vi "DF PROFINET IO GettingStarted Controller.vi"() -> ()   [LabVIEW 2019]
doc: "This VI shows how configured PROFINET devices can be accessed with a KUNBUS DF PROFINET IO interface card as Controller."
uses:
  <vilib>/KUNBUS GmbH/DF PROFINET IO/CS_PN_Profinet_StartStopMode.ctl
  <vilib>/KUNBUS GmbH/DF PROFINET IO/CS_PN_Controller_StartStopMode.ctl
  <vilib>/KUNBUS GmbH/DF PROFINET IO/CS_PN_Controller_WriteRecordReq.ctl
  <vilib>/KUNBUS GmbH/DF PROFINET IO/CS_PN_Controller_ReadRecordReq.ctl
  <vilib>/KUNBUS GmbH/DF PROFINET IO/CS_PN_Controller_AlarmClass.ctl
  <vilib>/Utility/error.llb/DialogType.ctl
panel:
  in  "Update time":u32=1 caption="(ms)"
  in  "Tab Control":enum32{"Process Data", "Read/Write Record Data"}(tab)
  out "Output data:":string
  out "Input data:":string
  in  "Modify output data:":string
  in  "Device List":i32(listbox)
  in  "Set output data":bool
  out "Description:":string
  in  "Get diagnostic data":bool
  in  "Get process data":bool
  in  "APDU status:":bool
  in  "Device status:":bool
  in  "Get modulediffblock":bool
  out "APDU status":u8 format="0x%02x"
  out "APDU status:":bool
  out "Device status":bool=TRUE
  out "Device status:":u8 format="0x%02x"
  in  "Output status 2":bool=TRUE caption="Status"
  out "Input status 2":u8 format="0x%02x"
  out "Input status":bool
  out "Output status 3":u8 format="0x%02x"
  out "Output status":bool
  out "Read record data:":string
  in  "Write record data:":string
  in  "Write Record":bool
  in  "Read Record":bool
  out "R/W Record Result":string
  out "Error out":errorcluster
  in  "Device":u16
  in  "Slot":u16
  in  "SubSlot":u16
  in  "Timeout":u32
  in  "Read data length":u32
  in  "Index":u16 format="%.0x"
  in  "Stop":bool
  in  "PROFINET Controller":refnum<visa-resource-name>
  # "Instructions:\n1. Read the Getting Started manual: Help >> KUNBUS GmbH >> DF PROFINET IO\n2. The PROFINET configuration needs to be downloaded to the DF PROFINET IO interface card using the configuration tool Configurator III\n3. Choose the DF PROFINET IO interface card from the VISA control \"PROFINET Controller\" and then start the VI"
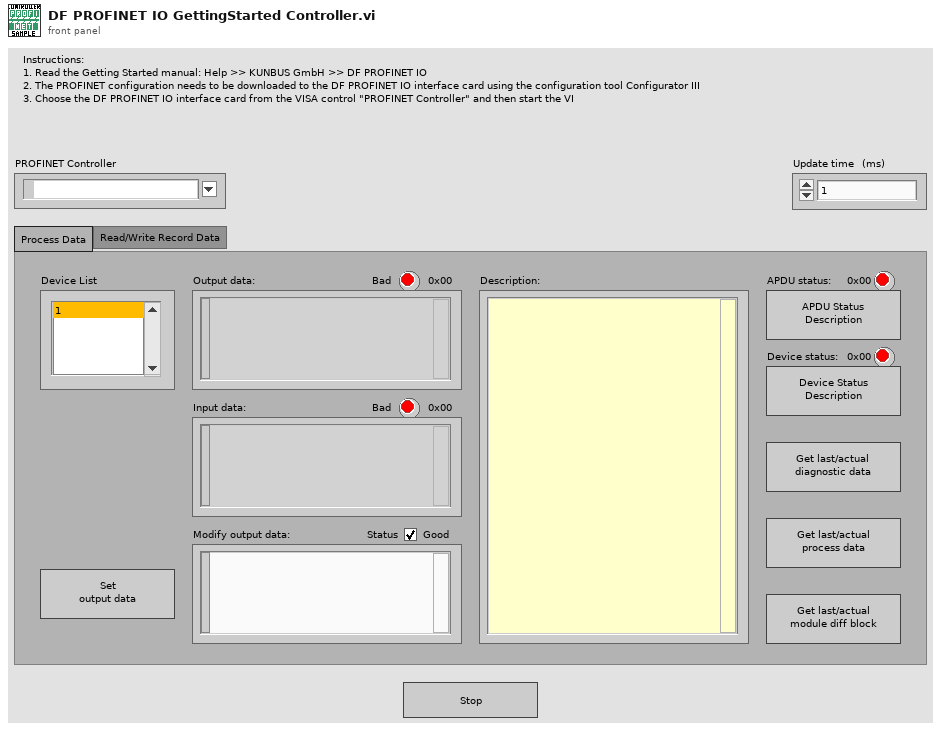
[diagram p1: front panel]
types:
  T1 = typedef "CS_PN_Controller_StartStopMode.ctl" = enum32{"Start Controller", "Stop Controller"}
  T2 = typedef "CS_PN_Profinet_StartStopMode.ctl" = enum32{"Start Controller", "Stop Controller", "Start Device", "Stop Device"}
  T3 = enum16{"APDU status", "Device status", "Diagnostic alarm data", "Process alarm data", "Module diff block"}
  T4 = typedef "CS_PN_Controller_AlarmClass.ctl" = u32
  T5 = typedef "CS_PN_Controller_AlarmData.ctl" = cluster{"Block type:":u16, "Block version:":u16, "Block length:":u16, "Alarm type:":T6, "API:":u32, "Slot number:":u16, "Subslot number:":u16, "Module ident number:":u32, "Submodule ident number:":u32, "Alarm specifier:":u16, "Alarm item:":u8[]}
  T6 = typedef "CS_PN_Controller_AlarmType.ctl" = u16
  T7 = typedef "CS_PN_Controller_ModDiffBlock.ctl" = cluster{"ARID:":u32, "Station name:":string, "Number of modules:":u32, "List of modules":T8[]}
  T8 = typedef "CS_PN_Controller_ModuleDiffBlockSlot.ctl" = cluster{"Slot number:":u32, "Module ident number:":u32, "Module state:":u32, "Number of submodules:":u32, "List of submodules":T9[]}
  T9 = typedef "CS_PN_Controller_ModuleDiffBlockSubslot.ctl" = cluster{"Subslot number:":u32, "Submodule ident number:":u32, "Submodule state:":u32}
  T10 = cluster{"Numeric":i32, "Output status":u8, "unsigned byte array":u8[]}
  T11 = cluster{"Numeric":i32, "Output status":u8, "unsigned byte array":u8[]}[]
  T12 = cluster{"APDU status":u8, "Device status":u8, "Input status":u8, "Input data":u8[], "Output status":u8, "Output data":u8[]}[]
  T13 = cluster{"APDU status":u8, "Device status":u8, "Input status":u8, "Input data":u8[], "Output status":u8, "Output data":u8[]}
  T14 = typedef "DialogType.ctl" = u16
  T15 = typedef "CS_PN_Controller_WriteRecordReq.ctl" = cluster{"Timeout:":u32, "Device:":u16, "Slot number:":u16, "Subslot number:":u16, "Index:":u16, "Record data:":u8[]}
  T16 = typedef "CS_PN_Controller_ReadRecordReq.ctl" = cluster{"Timeout:":u32, "Device:":u16, "Slot number:":u16, "Subslot number:":u16, "Index:":u16, "Data length:":u32}
  T17 = typedef "CS_PN_Controller_WriteRecordRes.ctl" = cluster{"Error code:":u8, "Error decode:":u8, "Error code 1:":u8, "Error code 2:":u8, "Add data 1:":u16, "Add data 2:":u16}
  T18 = typedef "CS_PN_Controller_ReadRecordRes.ctl" = cluster{"Error code:":u8, "Error decode:":u8, "Error code 1:":u8, "Error code 2:":u8, "Add data 1:":u16, "Add data 2:":u16, "Record data:":u8[]}
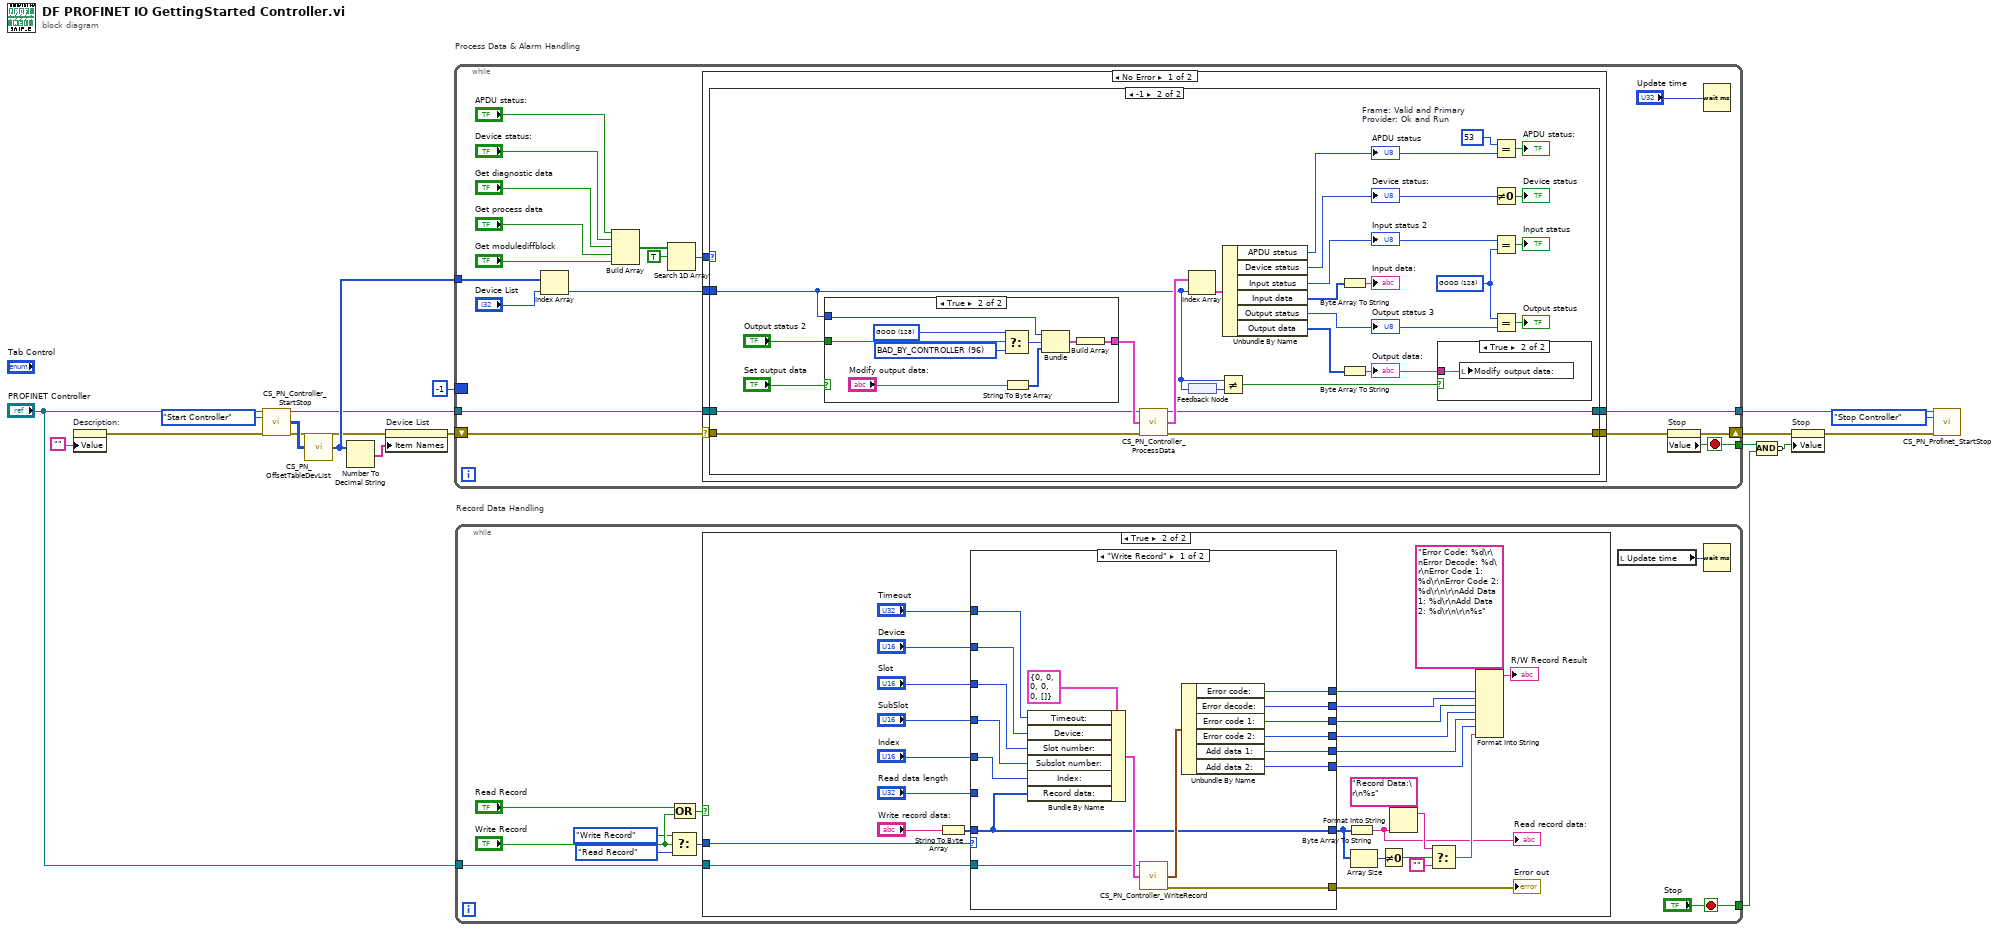
[diagram p0: block diagram]
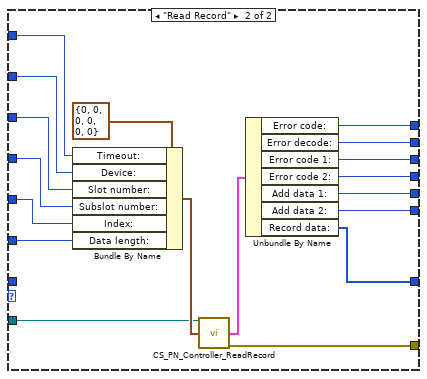
[diagram p3: hidden frame]
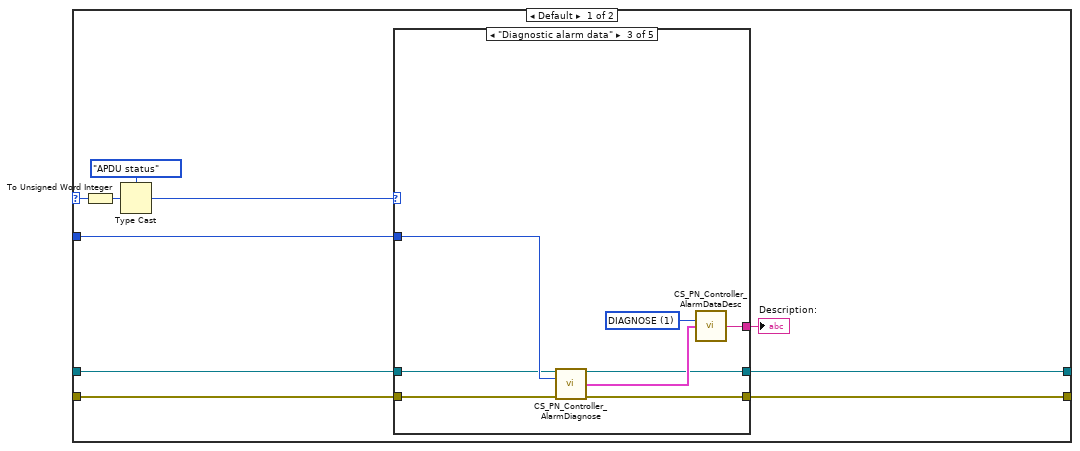
[diagram p4: hidden frame]
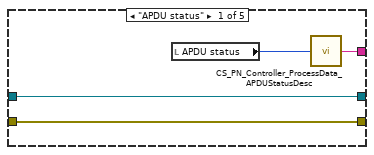
[diagram p5: hidden frame]
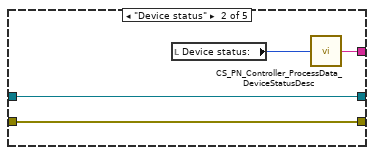
[diagram p6: hidden frame]
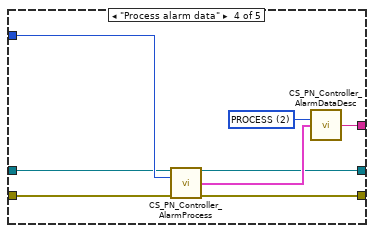
[diagram p7: hidden frame]
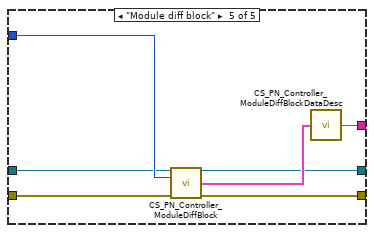
[diagram p8: hidden frame]
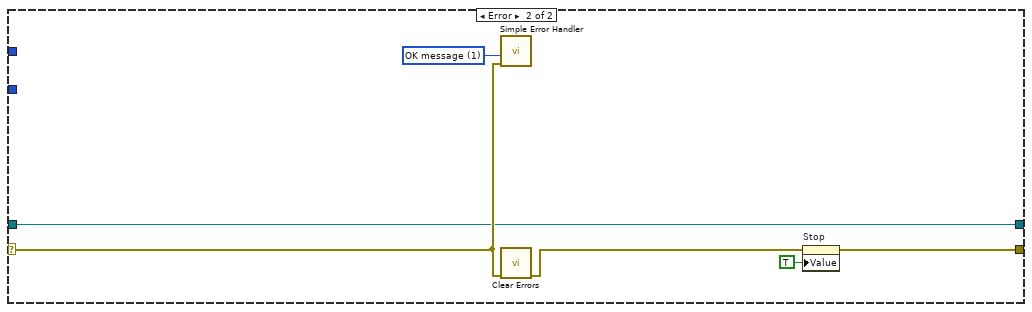
[diagram p11: hidden frame]
diagram:
  n1 = property on="Description:" class="Str"("Value"="") -> (error out=w9:errorcluster)  [unwired: 2 in, 1 out]
  n2 = call <vilib>:"CS_PN_Controller_StartStop.vi"("PN-Controller resource name"="PROFINET Controller", "Mode"=CS_PN_Controller_StartStopMode."Start Controller", "Error In"=w9) -> ("PN-Controller resource name out"=w7:refnum<visa-resource-name>, "Offset table info"=w13:i32[][], "Error Out"=w11:errorcluster)  [unwired: 9 in, 1 out]
  n3 = call <vilib>:"CS_PN_OffsetTableDevList.vi"("Offset table info"=w13) -> ("Device list"=w18:i32[])  [unwired: 14 in]
  n4 = Number To Decimal String(number=w18) -> (decimal integer string=w16:string[])  [unwired: 1 in]
  n5 = property on="Device List" class="LstBox (strict)"(error in=w11, "Item Names"=w16) -> (error out=w10:errorcluster)  [unwired: 1 in, 1 out]
  n6 = while "Process Data & Alarm Handling" {
    tunnel: w7 -> [w25]
    tunnel: [w35] -> w17
    tunnel: w18 -> [w36]
    border: -1 ("InitModifyOutputDataControl") -> [_]
    shift-right: [w20] -> w6
    shift-left: w10 -> [w22]
    tunnel: [w19] -> w3
    stop <- w19 stop-if-true
    n7 = Index Array(array=w36, index="Device List") -> (element=w34:i32)
    n8 = Build Array("APDU status:", "Device status:", "Get diagnostic data", "Get process data", "Get modulediffblock") -> (w30:bool[])
    n9 = Search 1D Array(1D array=w30, element=TRUE) -> (index of element=w24:i32)  [unwired: 1 in]
    n10 = case shown="No Error" w22 {
      selector: w22 -> [w37 w125]
      tunnel: [w42 w124] -> w35
      tunnel: w34 -> [w41 _]
      tunnel: w25 -> [w40 w124]
      tunnel: w24 -> [w39 _]
      tunnel: [w38 w122] -> w21
      frame No Error {
        n11 = case shown="-1" w39 {
          selector: w39 -> [w45 _]
          tunnel: w37 -> [w46 w109]
          tunnel: w40 -> [w47 w86]
          tunnel: [w43 w108] -> w38
          tunnel: [w44 w85] -> w42
          tunnel: w41 -> [w48 w87]
          frame Default {
            n12 = To Unsigned Word Integer(number=w45) -> (unsigned 16bit integer=w50:u16)
            n13 = Type Cast(type=T3."APDU status", x=w50) -> (*(type *) &x=w51:T3)
            n14 = case shown="\"Diagnostic alarm data\"" w51 {
              tunnel: w46 -> [w56 w59 w67 w75 w80]
              tunnel: w47 -> [w55 w60 w61 w74 w81]
              tunnel: [w56 w59 w65 w73 w79] -> w43
              tunnel: w48 -> [_ _ w68 w76 w83]
              tunnel: [w54 w58 w64 w71 w78] -> w52
              tunnel: [w55 w60 w63 w70 w77] -> w44
              frame "APDU status" {
                n15 = local read "APDU status"() -> (w53:u8)
                n16 = call <vilib>:"CS_PN_Controller_ProcessData_APDUStatusDesc.vi"("APDU Status"=w53) -> ("Description:"=w54:string)  [unwired: 14 in]
              }
              frame "Device status" {
                n17 = local read "Device status:"() -> (w57:u8)
                n18 = call <vilib>:"CS_PN_Controller_ProcessData_DeviceStatusDesc.vi"("Device Status"=w57) -> ("Description:"=w58:string)  [unwired: 14 in]
              }
              frame "Diagnostic alarm data" {
                w62 = T4 1 items=["DIAGNOSE"=1, "PROCESS"=2] ("AlarmClass")
                n19 = call <vilib>:"CS_PN_Controller_AlarmDiagnose.vi"("PN-Controller resource name"=w61, "Device"=w68, "Error In"=w67) -> ("PN-Controller resource name out"=w63:refnum<visa-resource-name>, "AlarmData"=w66:T5, "Error Out"=w65:errorcluster)  [unwired: 9 in, 1 out]
                n20 = call <vilib>:"CS_PN_Controller_AlarmDataDesc.vi"("AlarmClass"=w62, "AlarmData"=w66) -> ("Alarm data:"=w64:string)  [unwired: 13 in]
              }
              frame "Process alarm data" {
                w69 = T4 2 items=["DIAGNOSE"=1, "PROCESS"=2] ("AlarmClass")
                n21 = call <vilib>:"CS_PN_Controller_AlarmProcess.vi"("PN-Controller resource name"=w74, "Device"=w76, "Error In"=w75) -> ("PN-Controller resource name out"=w70:refnum<visa-resource-name>, "AlarmData"=w72:T5, "Error Out"=w73:errorcluster)  [unwired: 9 in, 1 out]
                n22 = call <vilib>:"CS_PN_Controller_AlarmDataDesc.vi"("AlarmClass"=w69, "AlarmData"=w72) -> ("Alarm data:"=w71:string)  [unwired: 13 in]
              }
              frame "Module diff block" {
                n23 = call <vilib>:"CS_PN_Controller_ModuleDiffBlock.vi"("PN-Controller resource name"=w81, "Device"=w83, "Error In"=w80) -> ("PN-Controller resource name out"=w77:refnum<visa-resource-name>, "ModuleDiffBlock"=w82:T7, "Error Out"=w79:errorcluster)  [unwired: 9 in, 1 out]
                n24 = call <vilib>:"CS_PN_Controller_ModuleDiffBlockDataDesc.vi"("ModuleDiffBlock"=w82) -> ("ModuelDiffBlock data:"=w78:string)  [unwired: 14 in]
              }
            }
            "Description:" <- w52
          }
          frame -1 {
            w84 = u8 128 items=["BAD"=0, "GOOD"=128] ("Output status")
            w89 = u8 53  # Frame: Valid and Primary Provider: Ok and Run
            n25 = case shown="True" "Set output data" {
              tunnel: [_ w117] -> w106
              tunnel: "Output status 2" -> [_ w115]
              tunnel: w87 -> [_ w111]
              frame False {
              }
              frame True {
                w116 = u8 128 items=["BAD"=0, "GOOD"=128] ("Output status")
                w114 = u8 96 items=["BAD_BY_SUBSLOT"=0, "BAD_BY_SLOT"=32, "BAD_BY_DEVICE"=64, "BAD_BY_CONTROLLER"=96, "GOOD"=128] ("Output status")
                n26 = Select(t=w116, s=w115, f=w114) -> (s? t:f=w113:u8)
                n27 = String To Byte Array(string="Modify output data:") -> (unsigned byte array=w112:u8[])
                n28 = Bundle("Numeric"=w111, "Output status"=w113, "unsigned byte array"=w112) -> (w118:T10)  [unwired: 1 in]
                n29 = Build Array(w118) -> (w117:T11)
              }
            }
            n30 = call <vilib>:"CS_PN_Controller_ProcessData.vi"("PN-Controller resource name"=w86, "Set process data"=w106, "Error In"=w109) -> ("PN-Controller resource name out"=w85:refnum<visa-resource-name>, "Get process data"=w107:T12, "Error Out"=w108:errorcluster)  [unwired: 9 in, 1 out]
            n31 = Index Array(array=w107, index=w87) -> (element=w103:T13)
            n32 = feedback #1() -> (w95:i32)
            n33 = feedback-in #1(w87) -> ()
            n34 = Not Equal?(x=w87, y=w95) -> (x != y?=w94:bool)
            n35 = Unbundle By Name(w103) -> ("APDU status"=w90:u8, "Device status"=w98:u8, "Input status"=w88:u8, "Input data"=w92:u8[], "Output status"=w91:u8, "Output data"=w93:u8[])
            "Device status:" <- w98
            "APDU status" <- w90
            "Input status 2" <- w88
            "Output status 3" <- w91
            n36 = Byte Array To String(unsigned byte array=w92) -> (string=→"Input data:":string)
            n37 = Byte Array To String(unsigned byte array=w93) -> (string=w99:string)
            "Output data:" <- w99
            n38 = case shown="True" w94 {
              tunnel: w99 -> [_ w110]
              frame False {
              }
              frame True {
                n39 = local write "Modify output data:"(w110) -> ()
              }
            }
            n40 = Equal?(x=w89, y=w90) -> (x = y?=→"APDU status:":bool)
            n41 = Not Equal To 0?(x=w98) -> (x != 0?=→"Device status":bool)
            n42 = Equal?(x=w88, y=w84) -> (x = y?=→"Input status":bool)
            n43 = Equal?(x=w84, y=w91) -> (x = y?=→"Output status":bool)
          }
        }
      }
      frame Error {
        w120 = T14 1 items=["no dialog", "OK message", "continue or stop message", "OK message + warnings", "continue/stop + warnings"] ("type of dialog (OK msg:1)")
        n44 = call <vilib>:"Simple Error Handler.vi"("type of dialog (OK msg:1)"=w120, "error in (no error)"=w125) -> ()  [unwired: 3 in, 5 out]
        n45 = call <vilib>:"Clear Errors.vi"("error in (no error)"=w125) -> ("error out"=w123:errorcluster)  [unwired: 5 in, 1 out]
        n46 = property on="Stop" class="Bool (strict)"(error in=w123, "Value"=TRUE ("Stop")) -> (error out=w122:errorcluster)  [unwired: 1 in, 1 out]
      }
    }
    n47 = property on="Stop" class="Bool (strict)"(error in=w21) -> (error out=w20:errorcluster, "Value"=w19:bool)  [unwired: 1 in, 1 out]
    n48 = Wait (ms)(milliseconds to wait="Update time") -> ()  [unwired: 1 out]
  }
  n49 = while "Record Data Handling" {
    tunnel: "PROFINET Controller" -> [w133]
    tunnel: ["Stop"] -> w4
    stop <- "Stop" stop-if-true
    n50 = Select(t=enum16{"Read Record", "Write Record"}."Write Record", s="Write Record", f=enum16{"Read Record", "Write Record"}."Read Record") -> (s? t:f=w126:enum16{"Read Record", "Write Record"})
    n51 = Compound Arithmetic op=OR("Read Record", "Write Record") -> (w130:bool)
    n52 = case shown="True" w130 {
      tunnel: w133 -> [_ w161]
      tunnel: w126 -> [_ w135]
      frame False {
      }
      frame True {
        n53 = String To Byte Array(string="Write record data:") -> (unsigned byte array=w137:u8[])
        n54 = case shown="\"Write Record\"" w135 {
          tunnel: w161 -> [w177 w194]
          tunnel: [w176 w192] -> w160
          tunnel: "Read data length" -> [_ w179]
          tunnel: "Timeout" -> [w167 w195]
          tunnel: "Device" -> [w166 w183]
          tunnel: "Slot" -> [w165 w182]
          tunnel: "SubSlot" -> [w164 w181]
          tunnel: "Index" -> [w163 w180]
          tunnel: [w173 w185] -> w139
          tunnel: [w172 w186] -> w152
          tunnel: [w171 w187] -> w151
          tunnel: [w170 w188] -> w150
          tunnel: [w169 w191] -> w149
          tunnel: [w168 w190] -> w148
          tunnel: [w162 w189] -> w145
          tunnel: w137 -> [w162 _]
          frame "Write Record" {
            n55 = Bundle By Name(cluster=T15 {"Timeout:"=0, "Device:"=0, "Slot number:"=0, "Subslot number:"=0, "Index:"=0, "Record data:"=[]} ("WriteRecord"), "Timeout:"=w167, "Device:"=w166, "Slot number:"=w165, "Subslot number:"=w164, "Index:"=w163, "Record data:"=w162) -> (w178:T15)
            n56 = call <vilib>:"CS_PN_Controller_WriteRecord.vi"("PN-Controller resource name"=w177, "WriteRecord"=w178) -> ("WriteRecordRet"=w174:T17, "Error Out"=w176:errorcluster)  [unwired: 10 in, 2 out]
            n57 = Unbundle By Name(w174) -> ("Error code:"=w173:u8, "Error decode:"=w172:u8, "Error code 1:"=w171:u8, "Error code 2:"=w170:u8, "Add data 1:"=w169:u16, "Add data 2:"=w168:u16)
          }
          frame "Read Record" {
            n58 = Bundle By Name(cluster=T16 {"Timeout:"=0, "Device:"=0, "Slot number:"=0, "Subslot number:"=0, "Index:"=0, "Data length:"=0} ("ReadRecord"), "Timeout:"=w195, "Device:"=w183, "Slot number:"=w182, "Subslot number:"=w181, "Index:"=w180, "Data length:"=w179) -> (w196:T16)
            n59 = call <vilib>:"CS_PN_Controller_ReadRecord.vi"("PN-Controller resource name"=w194, "ReadRecordReq"=w196) -> ("ReadRecordRes"=w184:T18, "Error Out"=w192:errorcluster)  [unwired: 10 in, 2 out]
            n60 = Unbundle By Name(w184) -> ("Error code:"=w185:u8, "Error decode:"=w186:u8, "Error code 1:"=w187:u8, "Error code 2:"=w188:u8, "Add data 1:"=w191:u16, "Add data 2:"=w190:u16, "Record data:"=w189:u8[])
          }
        }
        "Error out" <- w160
        n61 = Byte Array To String(unsigned byte array=w145) -> (string=w136:string)
        "Read record data:" <- w136
        n62 = Array Size(array=w145) -> (size(s)=w144:i32)
        n63 = Not Equal To 0?(x=w144) -> (x != 0?=w143:bool)
        n64 = Format Into String(format string="Record Data:\r\n%s", w136) -> (resulting string=w142:string)  [unwired: 2 in, 1 out]
        n65 = Select(t=w142, s=w143, f="") -> (s? t:f=w140:string)
        n66 = Format Into String(format string="Error Code: %d\r\nError Decode: %d\r\nError Code 1: %d\r\nError Code 2: %d\r\n\r\nAdd Data 1: %d\r\nAdd Data 2: %d\r\n\r\n%s", w139, w152, w151, w150, w149, w148, w140) -> (resulting string=→"R/W Record Result":string)  [unwired: 2 in, 1 out]
      }
    }
    n67 = local read "Update time"() -> (w134:u32)
    n68 = Wait (ms)(milliseconds to wait=w134) -> ()  [unwired: 1 out]
  }
  n69 = Compound Arithmetic op=AND(w3, w4) -> (invert w2:bool)
  n70 = property on="Stop" class="Bool (strict)"(error in=w6, "Value"=w2) -> (error out=w5:errorcluster)  [unwired: 1 in, 1 out]
  n71 = call <vilib>:"CS_PN_Profinet_StartStop.vi"("PN resource name"=w17, "Mode"=CS_PN_Profinet_StartStopMode."Stop Controller", "Error In"=w5) -> ()  [unwired: 9 in, 4 out]
